vi "Capture Screenshot.vi"(8 "error in (no error)":errorcluster, 10 "Overwrite? (Yes)":enum16{"Yes", "No", "Confirm"}(ring), 11 "Image Path":path) -> (0 "error out":errorcluster, 3 "dup Image Path":path)   [LabVIEW 2023]
doc: "Simulates a PrintScreen keystroke and saves the resulting screenshot to the location specified by <B>Image Path</B>. Acceptable extensions for the file are: .bmp, .gif, .jpeg, .jpg, .png, .tiff. Recommended extension is .png, as that is the extension Windows uses when normally capturing screenshots.\n\n<B>NOTE:</B> Using this VI will replace the contents of the clipboard with the screenshot itself."
uses:
  <vilib>/Utility/sysdir.llb/System Directory Type.ctl
  6bc9f4ba-f1e4-443d-910f-80dc0520f36e.vi
  <userlib>/_OpenG.lib/file/file.llb/File Exists - Scalar__ogtk.vi
  <userlib>/_OpenG.lib/file/file.llb/Strip Path Extension - Path__ogtk.vi
  <vilib>/Utility/error.llb/Error Cluster From Error Code.vi
  System.Drawing
  System.Windows.Forms
  <vilib>/ErrorRing/Error Ring.xnode
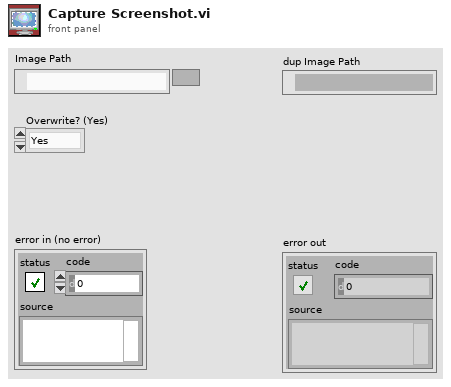
[diagram p1: front panel]
types:
  T1 = enum16{"Left Mouse Button", "Right Mouse Button", "Ctrl-Break", "Middle Mouse Button (3-button mice only)", "X1 mouse button (Win2k Only)", "X2 Mouse Button (Win2k Only)", "Undefined (1)", "BACKSPACE", "TAB", "Reserved (1)", "Reserved (2)", "CLEAR", "ENTER", "Undefined (2)", "Undefined (3)", "SHIFT", "CTRL", "ALT", "PAUSE", "CAPS LOCK", "IME Kana mode", "Undefined (4)", "IME Junja mode", "IME final mode", "IME Hanja mode", "IME Kanji mode", "Undefined    ", "ESC", "IME convert", "IME nonconvert", "IME accept", "IME mode change request", "SPACEBAR", "PAGE UP", "PAGE DOWN", "END", "HOME", "LEFT ARROW", "UP ARROW", "RIGHT ARROW", "DOWN ARROW", "SELECT", "PRINT", "EXECUTE", "PRINT SCREEN", "INS", "DEL", "HELP"}
  T2 = typedef "System Directory Type.ctl" = i32
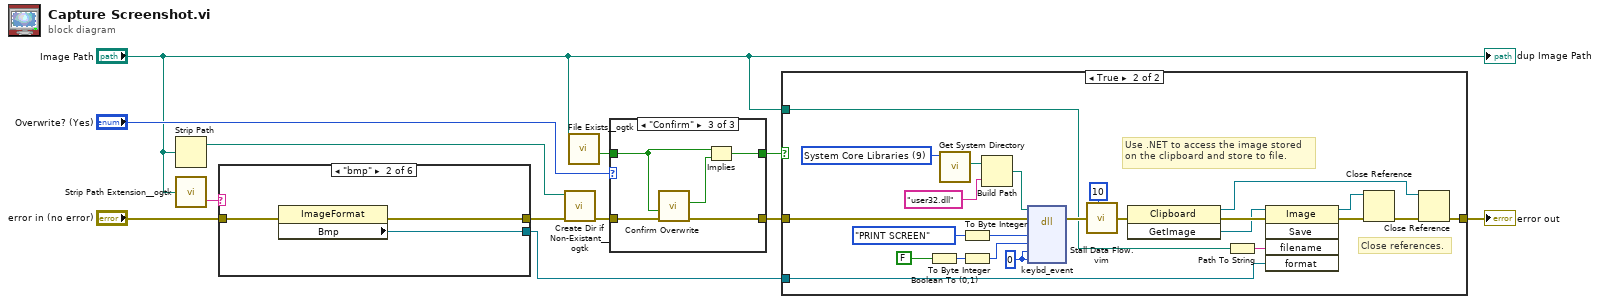
[diagram p0: block diagram]
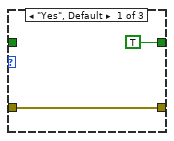
[diagram p3: hidden frame]
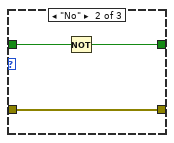
[diagram p4: hidden frame]
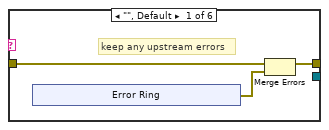
[diagram p5: hidden frame]
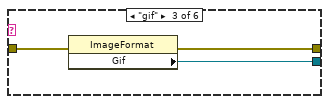
[diagram p6: hidden frame]
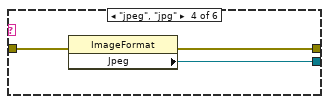
[diagram p7: hidden frame]
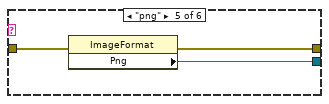
[diagram p8: hidden frame]
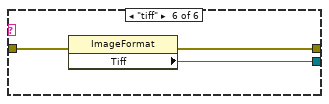
[diagram p9: hidden frame]
diagram:
  n1 = Strip Path(path="Image Path") -> (stripped path=w8:path)  [unwired: 1 out]
  n2 = call-poly <userlib>:"Strip Path Extension__ogtk.vi"("path"="Image Path") -> ("extension"=w9:string)  [unwired: 1 out]
  n3 = case shown="\"bmp\"" w9 {
    tunnel: "error in (no error)" -> [w14 w23 w26 w29 w32 w35]
    tunnel: [w15 w22 w25 w28 w31 w34] -> w10
    tunnel: [_ w21 w24 w27 w30 w33] -> w7
    frame "", Default {
      # "keep any upstream errors"
      n4 = xnode "Error Ring"() -> ("error out"=w13:errorcluster)
      n5 = Merge Errors(w14, w13) -> (w15:errorcluster)
    }
    frame "bmp" {
      n6 = property class="ImageFormat"(error in=w23) -> (error out=w22:errorcluster, "Bmp"=w21:refnum<k24>)  [unwired: 1 in, 1 out]
    }
    frame "gif" {
      n7 = property class="ImageFormat"(error in=w26) -> (error out=w25:errorcluster, "Gif"=w24:refnum<k24>)  [unwired: 1 in, 1 out]
    }
    frame "jpeg", "jpg" {
      n8 = property class="ImageFormat"(error in=w29) -> (error out=w28:errorcluster, "Jpeg"=w27:refnum<k24>)  [unwired: 1 in, 1 out]
    }
    frame "png" {
      n9 = property class="ImageFormat"(error in=w32) -> (error out=w31:errorcluster, "Png"=w30:refnum<k24>)  [unwired: 1 in, 1 out]
    }
    frame "tiff" {
      n10 = property class="ImageFormat"(error in=w35) -> (error out=w34:errorcluster, "Tiff"=w33:refnum<k24>)  [unwired: 1 in, 1 out]
    }
  }
  n11 = call <userlib>:"Create Dir if Non-Existant__ogtk.vi"("error in (no error)"=w10, "Directory Path"=w8) -> ("error out"=w2:errorcluster)  [unwired: 7 in, 2 out]
  n12 = call-poly <userlib>:"File Exists__ogtk.vi"("file path"="Image Path") -> ("exists"=w5:bool)  [unwired: 6 in, 1 out]
  n13 = case shown="\"Confirm\"" "Overwrite? (Yes)" {
    tunnel: w5 -> [_ w40 w42]
    tunnel: [TRUE w39 w43] -> w4
    tunnel: w2 -> [w36 w38 w45]
    tunnel: [w36 w38 w44] -> w1
    frame "Yes", Default {
    }
    frame "No" {
      n14 = Not(x=w40) -> (.not. x?=w39:bool)
    }
    frame "Confirm" {
      n15 = call "Confirm Overwrite"("error in (no error)"=w45, "Enable"=w42) -> ("error out"=w44:errorcluster, "Overwrite"=w41:bool)  [unwired: 8 in]
      n16 = Implies(1:w41, 2:w42) -> (0:w43:bool)
    }
  }
  n17 = case shown="True" w4 {
    tunnel: [w46 w70] -> w12
    tunnel: w1 -> [w46 w67]
    tunnel: w7 -> [_ w49]
    tunnel: "Image Path" -> [_ w47]
    frame False {
    }
    frame True {
      w57 = T2 9 items=["User Home"=0, "User Desktop"=1, "User Documents"=2, "User Application Data"=3, "User Preferences"=4, "User Temporary"=5, "Public Documents"=6, "Public Application Data"=7, "Public Preferences"=8, "Public Cache"=13, "System Core Libraries"=9, "System Installed Libraries"=10, "Application Files"=11, "Boot Volume Root"=12] ("system directory type")
      w58 = 0 ("Input Value")
      # "Close references."
      # "Use .NET to access the image stored\non the clipboard and store to file."
      n18 = Boolean To (0,1)(Boolean=FALSE ("T button?")) -> (0, 1=w62:i16)
      n19 = call <vilib>:"Get System Directory.vi"("system directory type"=w57) -> ("system directory"=w56:path)  [unwired: 10 in]
      n20 = To Byte Integer(number=T1."PRINT SCREEN" ("Keyboard Stroke 2")) -> (8bit integer=w63:i8)
      n21 = To Byte Integer(number=w62) -> (8bit integer=w59:i8)
      n22 = Build Path(base path=w56, name or relative path="user32.dll") -> (appended path=w54:path)
      n23 = dll-call lib="C:/Windows/System32/user32.dll" fn="keybd_event"(path in=w54, error in=w67, w63, w59, w58, w58) -> (error out=w69:errorcluster)  [unwired: 5 in, 2 out]
      n24 = call "Stall Data Flow.vim"("value in"=w69, "milliseconds to wait"=u32 10) -> ("value out"=w66:errorcluster)  [unwired: 1 out]
      n25 = invoke class="Clipboard" method="GetImage"(error in=w66) -> (reference out=w48:refnum<k24>, error out=w64:errorcluster, "GetImage"=w51:refnum<k24>)  [unwired: 2 in]
      n26 = Path To String(path=w47) -> (string=w50:string)
      n27 = invoke class="Image" method="Save"(reference=w51, error in=w64, "filename"=w50, "format"=w49) -> (reference out=w52:refnum<k24>, error out=w68:errorcluster)  [unwired: 1 in, 3 out]
      n28 = Close Reference(reference=w52, error in (no error)=w68) -> (error out=w65:errorcluster)
      n29 = Close Reference(reference=w48, error in (no error)=w65) -> (error out=w70:errorcluster)
    }
  }
  "error out" <- w12
  "dup Image Path" <- "Image Path"
